vi "Open.vi"(8 "error in (no error)":errorcluster, 11 "TCP Comm":T1) -> (0 "error out":errorcluster)   [LabVIEW 2020, in "TCP Comms.lvlib"]
uses:
  TCP Comms.lvlib
  TCP Comm.ctl
  Ref Data.ctl
  State.ctl
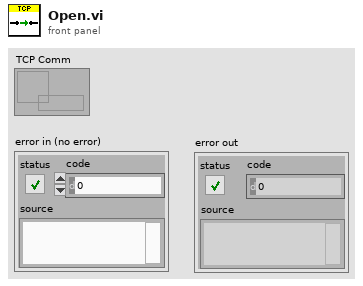
[diagram p1: front panel]
types:
  T1 = typedef "TCP Comms.lvlib/TCP Comm.ctl" = refnum<data-value>
  T2 = typedef "TCP Comms.lvlib/Ref Data.ctl" = cluster{"TCP":refnum<k5>, "State":T3, "Server":bool, "Host":string, "Port":u16, "Listener":refnum<k5>, "Start":bool, "Disconnect":bool, "TCP Valid":bool, "TLS Enabled":bool, "Immutable TLS":refnum<k36>, "Certificate DN":string}
  T3 = typedef "TCP Comms.lvlib/State.ctl" = enum16{"Idle", "Starting", "Connecting", "Connected", "Disconnecting", "Stopped"}
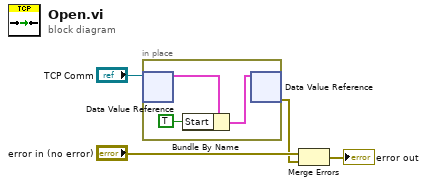
[diagram p0: block diagram]
diagram:
  n1 = in-place {
    n2 = in-place-dvr #1("TCP Comm") -> (w7:T2)  [unwired: 1 out]
    n3 = Bundle By Name(cluster=w7, "Start"=TRUE) -> (w6:T2)
    n4 = in-place-dvr #1(w6) -> (w2:errorcluster)  [unwired: 1 out]
  }
  n5 = Merge Errors("error in (no error)", w2) -> (→"error out":errorcluster)
